vi "get joystick settings.vi"(8 "error in (no error)":errorcluster, 10 "joystick_settings":T1, 11 "id":i32) -> (0 "error out":errorcluster, 2 "joystick_settings out":T1, 3 "function return":i32)   [LabVIEW 2012, in "libximc.lvlib"]
doc: "result_t XIMC_API get_joystick_settings (device_t id, joystick_settings_t* joystick_settings);"
uses:
  libximc.lvlib
  libximc.dll
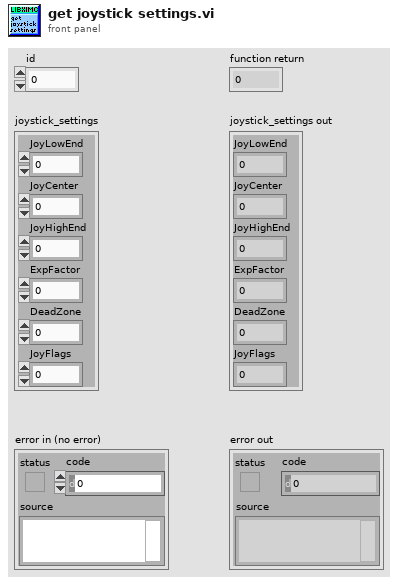
[diagram p1: front panel]
types:
  T1 = cluster{"JoyLowEnd":u32, "JoyCenter":u32, "JoyHighEnd":u32, "ExpFactor":u32, "DeadZone":u32, "JoyFlags":u32}
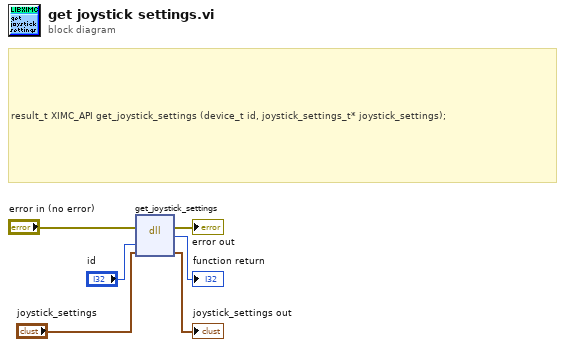
[diagram p0: block diagram]
diagram:
  # "result_t XIMC_API get_joystick_settings (device_t id, joystick_settings_t* joystick_settings);"
  n1 = dll-call lib="C:/Users/Vasily/Att_examples/LabVIEW_example/libximc.*" fn="get_joystick_settings"(error in="error in (no error)", "id"="id", "joystick_settings"="joystick_settings") -> (error out=→"error out":errorcluster, →"function return":i32, "joystick_settings"=→"joystick_settings out":T1)  [unwired: 3 in, 1 out]
